vi "Wait for Trigger State_Actions.vi"(9 "Pre-Trigger Samples":u16, 10 "Acq Hold=0?":bool=TRUE, 11 "Reference Trigger":bool=TRUE) -> (3 "State Execution Outputs":T1)   [LabVIEW 2012]
uses:
  State Execution Output.ctl
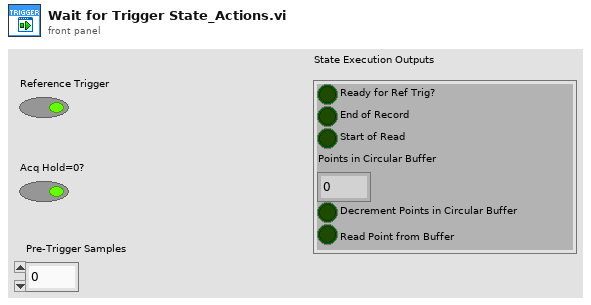
[diagram p1: front panel]
types:
  T1 = typedef "State Execution Output.ctl" = cluster{"Ready for Ref Trig?":bool, "End of Record":bool, "Start of Read":bool, "Points in Circular Buffer":u16, "Decrement Points in Circular Buffer":bool, "Read Point from Buffer":bool}
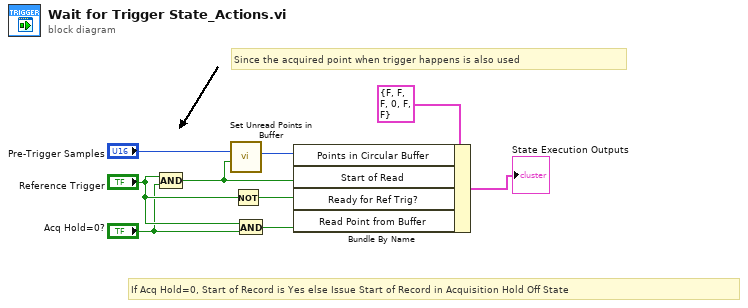
[diagram p0: block diagram]
diagram:
  # "If Acq Hold=0, Start of Record is Yes else Issue Start of Record in Acquisition Hold Off State"
  # "Since the acquired point when trigger happens is also used"
  n1 = Compound Arithmetic op=AND("Reference Trigger", "Acq Hold=0?") -> (w2:bool)
  n2 = call "Set Unread Points in Buffer.vi"("Set"=w2, "Value"="Pre-Trigger Samples") -> ("Value"=w8:u16)  [unwired: 9 in]
  n3 = Not(x="Reference Trigger") -> (.not. x?=w9:bool)
  n4 = And(x="Reference Trigger", y="Acq Hold=0?") -> (x .and. y?=w7:bool)
  n5 = Bundle By Name(cluster=T1 {"Ready for Ref Trig?"=FALSE, "End of Record"=FALSE, "Start of Read"=FALSE, "Points in Circular Buffer"=0, "Decrement Points in Circular Buffer"=FALSE, "Read Point from Buffer"=FALSE} ("State Execution Outputs"), "Points in Circular Buffer"=w8, "Start of Read"=w2, "Ready for Ref Trig?"=w9, "Read Point from Buffer"=w7) -> (→"State Execution Outputs":T1)
